vi "absCalcPlot_IV.vi"(4 "crd":dbl, 5 "file path (dialog if empty)":path, 6 "Cell Calibration, mV/mW":dbl=600000.0, 7 "save?":bool, 8 "Error In":errorcluster, 9 "PD Values":cluster{dbl, dbl, dbl, dbl}, 10 "bkg values":cluster{dbl, dbl, dbl, dbl}, 11 "Mic Values":cluster{dbl, dbl, dbl, dbl}) -> (0 "Error Out":errorcluster, 1 "aae":dbl, 2 "b_abs/ext ts":cluster{dbl, dbl, dbl, dbl, "crd":dbl}, 3 "Spectrum":cluster{dbl[], "Best Power Fit":dbl[]}[](graph))   [LabVIEW 2011]
uses:
  <vilib>/Analysis/NI_AALPro.lvlib
panel:
  out "output cluster":cluster{i32[], "Best Power Fit":dbl[]}
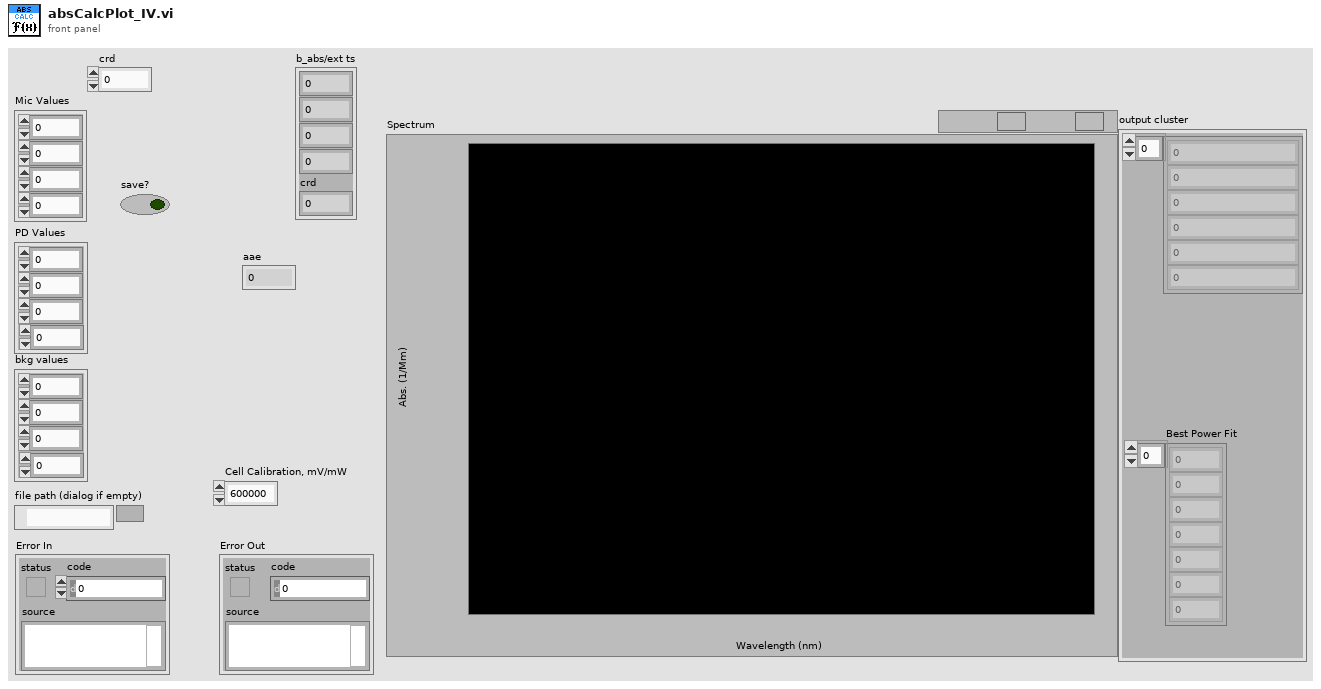
[diagram p1: front panel]
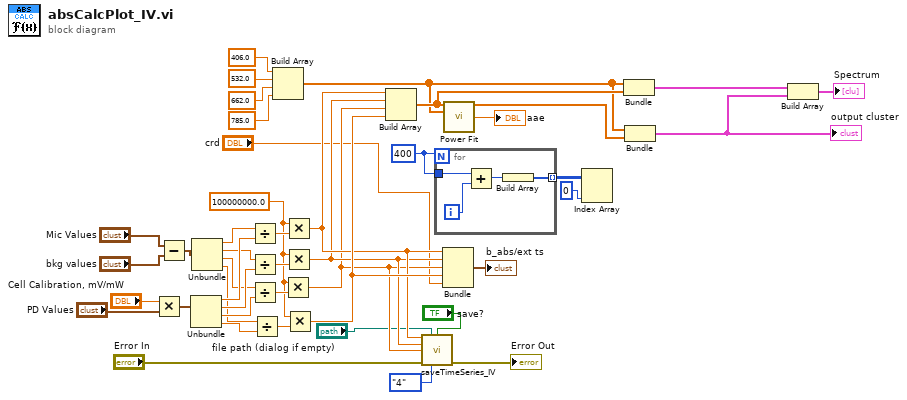
[diagram p0: block diagram]
diagram:
  w13 = 100000000.0 ("element")
  w28 = 400
  n1 = Multiply(x="Cell Calibration, mV/mW", y="PD Values") -> (x*y=w38:cluster{dbl, dbl, dbl, dbl})
  n2 = Subtract(x="Mic Values", y="bkg values") -> (x-y=w30:cluster{dbl, dbl, dbl, dbl})
  n3 = Unbundle(w38) -> (w39:dbl, w40:dbl, w41:dbl, w14:dbl)
  n4 = Unbundle(w30) -> (w33:dbl, w34:dbl, w35:dbl, w15:dbl)
  n5 = Divide(x=w33, y=w39) -> (x/y=w22:dbl)
  n6 = Divide(x=w34, y=w40) -> (x/y=w21:dbl)
  n7 = Divide(x=w35, y=w41) -> (x/y=w20:dbl)
  n8 = Divide(x=w15, y=w14) -> (x/y=w16:dbl)
  n9 = Build Array(406.0 ("element"), 532.0 ("element"), 662.0 ("element"), 785.0 ("element")) -> (w18:dbl[])
  n10 = Multiply(x=w13, y=w20) -> (x*y=w8:dbl)
  n11 = Multiply(x=w13, y=w22) -> (x*y=w10:dbl)
  n12 = Multiply(x=w13, y=w21) -> (x*y=w9:dbl)
  n13 = Multiply(x=w13, y=w16) -> (x*y=w11:dbl)
  n14 = Build Array(w10, w9, w8, w11) -> (w19:dbl[])
  n15 = call "saveTimeSeries_IV.vi"("1"=w10, "file path (dialog if empty)"="file path (dialog if empty)", "save?"="save?", "2"=w9, "3"=w8, "Error In"="Error In", "Number of Data Series"=enum16{"1", "2", "3", "4"}."4") -> ("Error Out"=→"Error Out":errorcluster)  [unwired: 8 in]
  n16 = for {
    N: w28 -> [_]
    tunnel: w28 -> [w47]
    tunnel: [w45] -> w26 mode=indexing
    i -> [w48]
    n17 = Add(x=w47, y=w48) -> (x+y=w46:i32)
    n18 = Build Array(w46) -> (w45:i32[])
  }
  n19 = Bundle(w10, w9, w8, w11, "crd"="crd") -> (→"b_abs/ext ts":cluster{dbl, dbl, dbl, dbl, "crd":dbl})  [unwired: 1 in]
  n20 = call <vilib>:"Power Fit.vi"("Y"=w19, "X"=w18) -> ("Best Power Fit"=w27:dbl[], "power"=→"aae":dbl)  [unwired: 8 in, 4 out]
  n21 = Index Array(array=w26, index (col)=0 ("index (row)")) -> ()  [unwired: 1 in, 1 out]
  n22 = Bundle(w18, w19) -> (w17:cluster{dbl[], dbl[]})  [unwired: 1 in]
  n23 = Bundle(w18, "Best Power Fit"=w27) -> (w25:cluster{dbl[], "Best Power Fit":dbl[]})  [unwired: 1 in]
  "output cluster" <- w25
  n24 = Build Array(w17, w25) -> (→"Spectrum":cluster{dbl[], "Best Power Fit":dbl[]}[])
